vi "TCP Initialize Client - Local.vi"(8 "error in (no error)":errorcluster, 10 "timeout ms (60000)":i32=60000, 11 "Service Name":string) -> (0 "error out":errorcluster, 3 "connection ID Out":refnum<k5>)   [LabVIEW 2016, in "SLL Easy API via TCP.lvclass"]
doc: "Opens a TCP Connection for the Service Name provided."
uses:
  SLL Easy API via TCP.lvclass
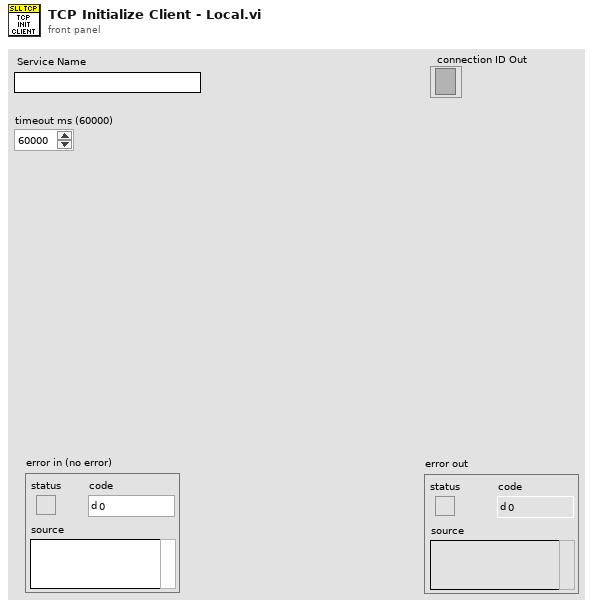
[diagram p1: front panel]
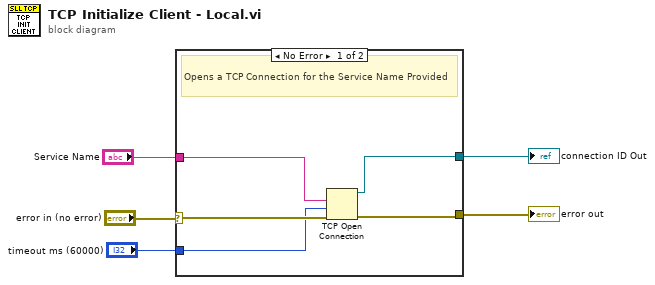
[diagram p0: block diagram]
diagram:
  n1 = case shown="No Error" "error in (no error)" {
    selector: "error in (no error)" -> [w10 w11]
    tunnel: [w9 w11] -> w4
    tunnel: "Service Name" -> [w8 _]
    tunnel: [w7 _] -> w2
    tunnel: "timeout ms (60000)" -> [w6 _]
    frame No Error {
      # "Opens a TCP Connection for the Service Name Provided"
      n2 = TCP Open Connection(remote port or service name=w8, timeout ms (60000)=w6, error in (no error)=w10) -> (connection ID=w7:refnum<k5>, error out=w9:errorcluster)  [unwired: 2 in]
    }
    frame Error {
    }
  }
  "error out" <- w4
  "connection ID Out" <- w2
